vi "TestNewPathGeneration.vi"() -> ()   [LabVIEW 2020]
panel:
  out "Results":cluster{"Boolean":bool, "PathOut":path}[](array[cluster])=[{"Boolean"=TRUE, "PathOut"=path "c:/temp/Name_class"}, {"Boolean"=TRUE, "PathOut"=path "c:/temp/Name_class"}, {"Boolean"=FALSE, "PathOut"=path "c:/temp/Name_interface/Hello_class"}]
  in  "UnitTesting":T1(array[cluster])=[{"NewPath"=path "c:/temp", "OldPath"=path "c:/temp", "NewName"="Name", "OldName"="Name", "NewSuffix"="_class", "OldSuffix"="_interface", "PathOut"=path "c:/temp/Name_class"}, {"NewPath"=path "c:/temp/Name_interface", "OldPath"=path "c:/temp/Name_interface", "NewName"="Name", "OldName"="Name", "NewSuffix"="_class", "OldSuffix"="_interface", "PathOut"=path "c:/temp/Name_class"}, {"NewPath"=path "c:/temp/Name_class", "OldPath"=path "c:/temp/Name_class", "NewName"="Hello", "OldName"="Name", "NewSuffix"="_class", "OldSuffix"="_class", "PathOut"=path "c:/temp/Hello_class"}]
  in  "_NewClassPath":path=path "c:/Temp" caption="New Class Folder"
  in  "_UseClassSuffix":string="_class" caption="Class Folder Suffix"
  in  "_NewClassName":string="Test" caption="New Class Name"
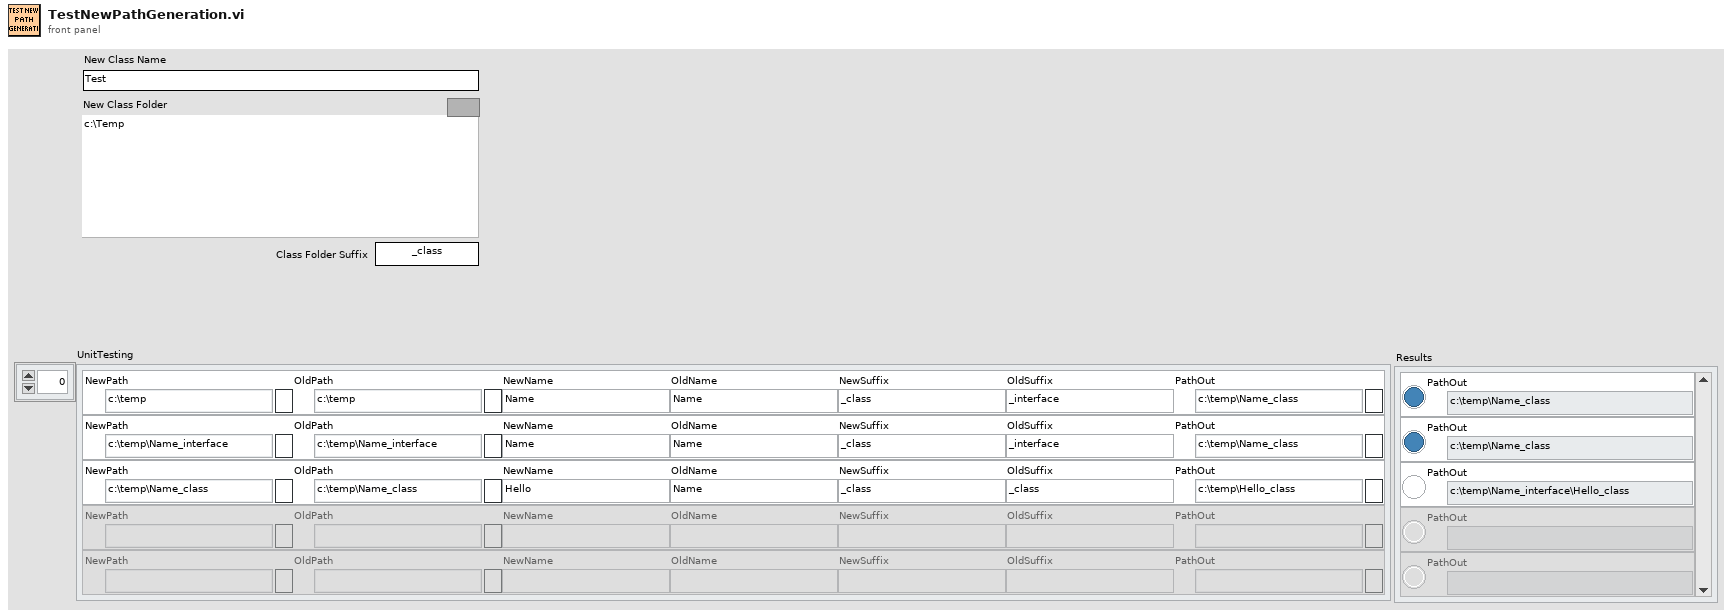
[diagram p1: front panel]
types:
  T1 = cluster{"NewPath":path, "OldPath":path, "NewName":string, "OldName":string, "NewSuffix":string, "OldSuffix":string, "PathOut":path}[]
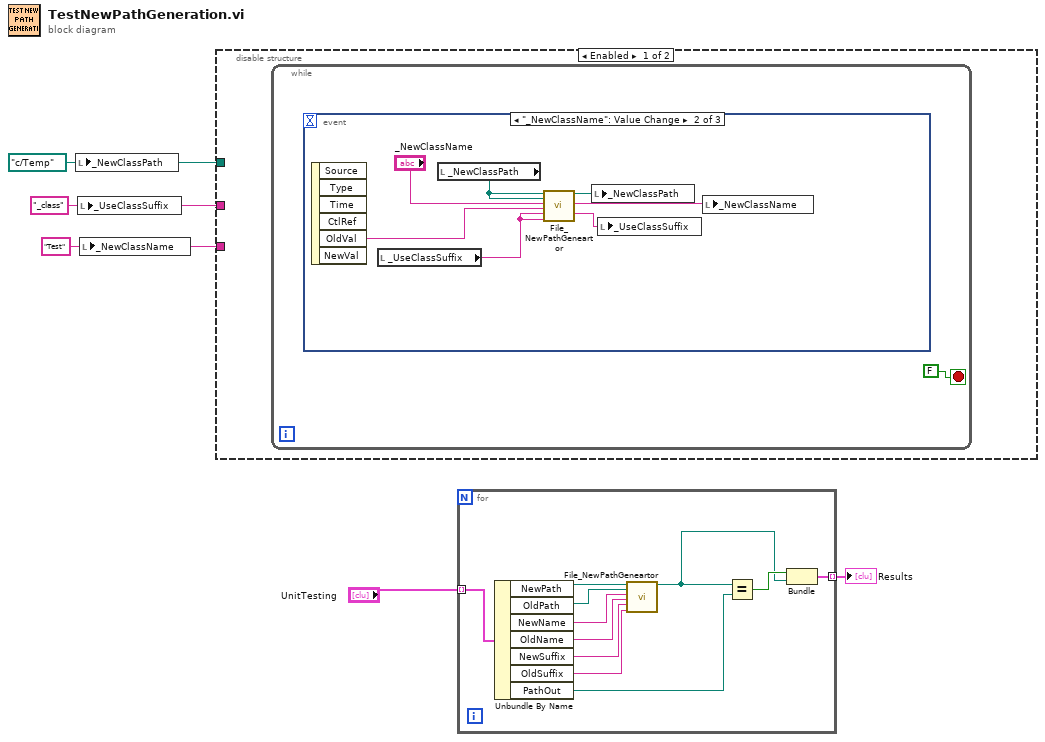
[diagram p0: block diagram]
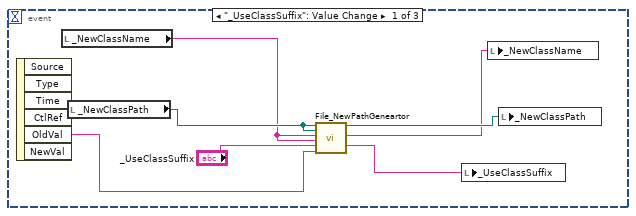
[diagram p2: hidden frame]
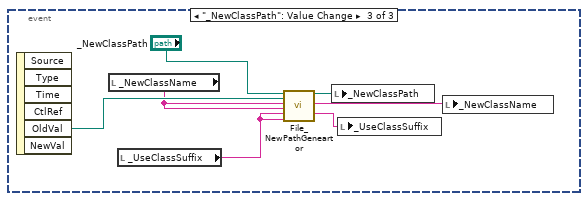
[diagram p3: hidden frame]
diagram:
  w2 = "Test" ("_NewClassName")
  w1 = "_class" ("_UseClassSuffix")
  w3 = path "c:/Temp" ("_NewClassPath")
  n1 = local write "_NewClassPath"(w3) -> ()
  n2 = local write "_UseClassSuffix"(w1) -> ()
  n3 = local write "_NewClassName"(w2) -> ()
  n4 = disable-structure shown="Enabled" {
    disable-tunnel: w3 -> [_ _]
    disable-tunnel: w2 -> [_ _]
    disable-tunnel: w1 -> [_ _]
    frame Enabled {
      n5 = while {
        stop <- FALSE stop-if-true
        n6 = event shown="[1] \"_NewClassName\": Value Change" {
          selector: _ -> [_ _ _]
          dyn-events: _ -> [_ _ _]
          timeout: _ -> [_ _ _]
          event "_UseClassSuffix": Value Change {
            n7 = event-data() -> ("OldVal"=w7:string)  [unwired: 1 in, 5 out]
            n8 = local read "_NewClassName"() -> (w9:string)
            n9 = local read "_NewClassPath"() -> (w10:path)
            n10 = call <resource>:"File_NewPathGeneartor.vi"("NewPath"=w10, "OldPath"=w10, "NewName"=w9, "OldName"=w9, "NewSuffix"="_UseClassSuffix", "OldSuffix"=w7) -> ("PathOut"=w12:path, "NameOut"=w11:string, "SuffixOut"=w13:string)  [unwired: 11 in]
            n11 = local write "_UseClassSuffix"(w13) -> ()
            n12 = local write "_NewClassName"(w11) -> ()
            n13 = local write "_NewClassPath"(w12) -> ()
          }
          event "_NewClassName": Value Change {
            n14 = event-data() -> ("OldVal"=w19:string)  [unwired: 1 in, 5 out]
            n15 = local read "_UseClassSuffix"() -> (w18:string)
            n16 = local read "_NewClassPath"() -> (w17:path)
            n17 = call <resource>:"File_NewPathGeneartor.vi"("NewPath"=w17, "OldPath"=w17, "NewName"="_NewClassName", "OldName"=w19, "NewSuffix"=w18, "OldSuffix"=w18) -> ("PathOut"=w16:path, "NameOut"=w15:string, "SuffixOut"=w14:string)  [unwired: 11 in]
            n18 = local write "_NewClassPath"(w16) -> ()
            n19 = local write "_UseClassSuffix"(w14) -> ()
            n20 = local write "_NewClassName"(w15) -> ()
          }
          event "_NewClassPath": Value Change {
            n21 = event-data() -> ("OldVal"=w22:path)  [unwired: 1 in, 5 out]
            n22 = local read "_NewClassName"() -> (w21:string)
            n23 = local read "_UseClassSuffix"() -> (w27:string)
            n24 = call <resource>:"File_NewPathGeneartor.vi"("NewPath"="_NewClassPath", "OldPath"=w22, "NewName"=w21, "OldName"=w21, "NewSuffix"=w27, "OldSuffix"=w27) -> ("PathOut"=w26:path, "NameOut"=w25:string, "SuffixOut"=w24:string)  [unwired: 11 in]
            n25 = local write "_NewClassPath"(w26) -> ()
            n26 = local write "_UseClassSuffix"(w24) -> ()
            n27 = local write "_NewClassName"(w25) -> ()
          }
        }
      }
    }
    frame Disabled {
    }
  }
  n28 = for {
    tunnel: "UnitTesting" -> [w38] mode=indexing
    tunnel: [w28] -> w4 mode=indexing
    n29 = Unbundle By Name(w38) -> ("NewPath"=w37:path, "OldPath"=w36:path, "NewName"=w35:string, "OldName"=w34:string, "NewSuffix"=w33:string, "OldSuffix"=w32:string, "PathOut"=w31:path)
    n30 = call <resource>:"File_NewPathGeneartor.vi"("NewPath"=w37, "OldPath"=w36, "NewName"=w35, "OldName"=w34, "NewSuffix"=w33, "OldSuffix"=w32) -> ("PathOut"=w29:path)  [unwired: 11 in, 2 out]
    n31 = Equal?(x=w29, y=w31) -> (x = y?=w30:bool)
    n32 = Bundle(w30, "PathOut"=w29) -> (w28:cluster{bool, "PathOut":path})  [unwired: 1 in]
  }
  "Results" <- w4
